vi "CAlex2_InitAll_ExtWt.vi"(7 "CAlexVersion":T1=enum."Mobile", 8 "error in (no error)":errorcluster, 9 "ExtraWeight(kg)":cluster{"Thigh":dbl, "Shank":dbl}, 10 "LegProperties":T2={"BodyDim"={"ThighLt (m)"=0.4, "ShankLt (m)"=0.41, "HipWd (m)"=0.32}, "BodyWt"={"Thigh (kg)"=0.0, "Shank (kg)"=0.0}, "Cuff Loc"={"HipCuffWd (m)"=0.4, "HipCuffHt (m)"=0.1, "HipFwdShift (m)"=0.0, "ThighToKnee (m)"=0.25, "ThighCuffDist (m)"=0.0, "ShankToKnee (m)"=0.15}}, 11 "CAlex2 in":refnum<class "CAlex2.lvclass">) -> (0 "error out":errorcluster, 3 "CAlex2 out":refnum<class "CAlex2.lvclass">)   [LabVIEW 2016, in "CAlex2.lvclass"]
uses:
  CAlex2.lvclass
  C:/Users/randh/Desktop/CABLE-LABVIEW/CALEX/CAlex2-controller/Classes/SerialChain/SerialChain.lvclass
  TypeDef/LowerBodyDim.ctl
  TypeDef/CAlexVersion.ctl
  SerialChain/TypeDef/xyzO.ctl
  <vilib>/Analysis/Matrix/Datatypes/RealMatrix.ctl
  CAlex2.lvclass/CAlex2.ctl
  SerialChain/SerialChain.lvclass
  <vilib>/Analysis/Matrix/NI_Matrix.lvlib
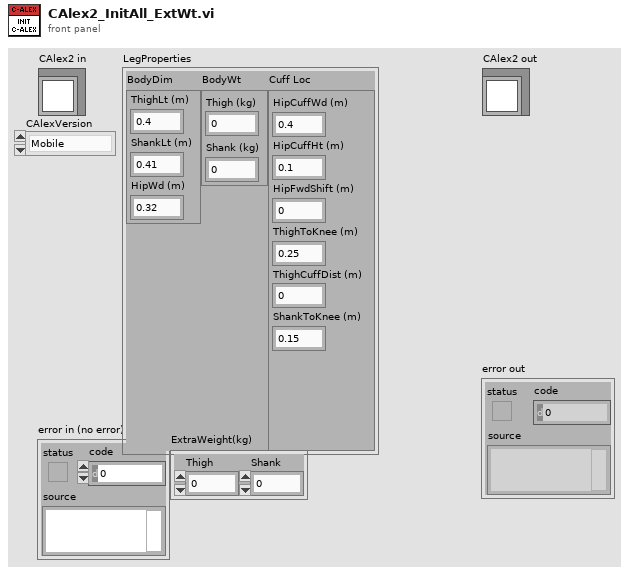
[diagram p1: front panel]
types:
  T1 = typedef "CAlex2.lvclass/CAlexVersion.ctl" = enum16{"Bilateral_Squat", "Treadmill", "Mobile"}
  T2 = typedef "CAlex2.lvclass/LowerBodyDim.ctl" = cluster{"BodyDim":cluster{"ThighLt (m)":dbl, "ShankLt (m)":dbl, "HipWd (m)":dbl}, "BodyWt":cluster{"Thigh (kg)":dbl, "Shank (kg)":dbl}, "Cuff Loc":cluster{"HipCuffWd (m)":dbl, "HipCuffHt (m)":dbl, "HipFwdShift (m)":dbl, "ThighToKnee (m)":dbl, "ThighCuffDist (m)":dbl, "ShankToKnee (m)":dbl}}
  T3 = typedef "NI_Matrix.lvlib/RealMatrix.ctl" = dbl[][]
  T4 = typedef "SerialChain.lvclass/xyzO.ctl" = enum16{"X", "Y", "Z", "O"}
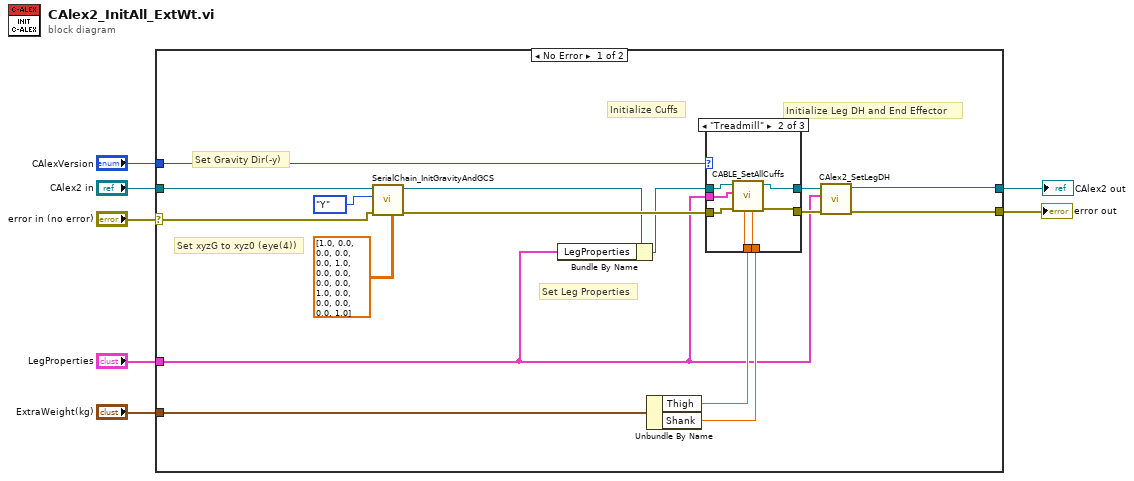
[diagram p0: block diagram]
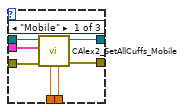
[diagram p2: hidden frame]
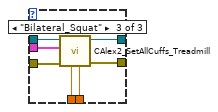
[diagram p3: hidden frame]
diagram:
  n1 = case shown="No Error" "error in (no error)" {
    selector: "error in (no error)" -> [w15 w46]
    tunnel: [w14 w46] -> w6
    tunnel: [w20 w45] -> w5
    tunnel: "CAlex2 in" -> [w22 w45]
    tunnel: "ExtraWeight(kg)" -> [w10 _]
    tunnel: "LegProperties" -> [w9 _]
    tunnel: "CAlexVersion" -> [w8 _]
    frame No Error {
      # "Initialize Leg DH and End Effector"
      # "Initialize Cuffs"
      # "Set Leg Properties"
      # "Set xyzG to xyz0 (eye(4))"
      # "Set Gravity Dir(-y)"
      n2 = call "SerialChain_InitGravityAndGCS.vi"("Trans_Gto0 (eye(4))"=T3 [[1.0, 0.0, 0.0, 0.0], [0.0, 1.0, 0.0, 0.0], [0.0, 0.0, 1.0, 0.0], [0.0, 0.0, 0.0, 1.0]] ("Trans_0toG"), "error in (no error)"=w15, "Gravity Axis in G (Z)"=xyzO."Y" ("Gravity Axis"), "SerialChain in"=w22) -> ("error out"=w18:errorcluster, "SerialChain out"=w17:refnum<class "CAlex2.lvclass">)  [unwired: 6 in]
      n3 = Bundle By Name(cluster=w17, "LegProperties"=w9) -> (w16:refnum<class "CAlex2.lvclass">)
      n4 = Unbundle By Name(w10) -> ("Thigh"=w12:dbl, "Shank"=w11:dbl)
      n5 = case shown="\"Treadmill\"" w8 {
        tunnel: [w30 w32 w44] -> w21
        tunnel: [w29 w33 w43] -> w19
        tunnel: w18 -> [w28 w34 w42]
        tunnel: w16 -> [w27 w31 w41]
        tunnel: w12 -> [w26 w37 w40]
        tunnel: w11 -> [w25 w36 w39]
        tunnel: w9 -> [w24 w35 w38]
        frame "Mobile" {
          n6 = call-dynamic "CAlex2_SetAllCuffs_Mobile.vi"("ShankExtraWeight"=w25, "ThighExtraWeight"=w26, "error in (no error)"=w28, "LegProperty"=w24, "CAlex2 in"=w27) -> ("error out"=w29:errorcluster, "CAlex2 out"=w30:refnum<class "CAlex2.lvclass">)  [unwired: 5 in]
        }
        frame "Treadmill" {
          n7 = call-dynamic "CABLE_SetAllCuffs.vi"("ShankExtraWeight"=w36, "ThighExtraWeight"=w37, "error in (no error)"=w34, "LegProperty"=w35, "CAlex2 in"=w31) -> ("error out"=w33:errorcluster, "CAlex2 out"=w32:refnum<class "CAlex2.lvclass">)  [unwired: 5 in]
        }
        frame "Bilateral_Squat" {
          n8 = call-dynamic "CAlex2_SetAllCuffs_Treadmill.vi"("ShankExtraWeight"=w39, "ThighExtraWeight"=w40, "error in (no error)"=w42, "LegProperty"=w38, "CAlex2 in"=w41) -> ("error out"=w43:errorcluster, "CAlex2 out"=w44:refnum<class "CAlex2.lvclass">)  [unwired: 5 in]
        }
      }
      n9 = call "CAlex2_SetLegDH.vi"("error in (no error)"=w19, "ArmProperty"=w9, "CAlex2 in"=w21) -> ("error out"=w14:errorcluster, "CAlex2 out"=w20:refnum<class "CAlex2.lvclass">)  [unwired: 7 in]
    }
    frame Error {
    }
  }
  "error out" <- w6
  "CAlex2 out" <- w5
